vi "pwm_LED.vi"() -> ()   [LabVIEW 2011]
uses:
  <vilib>/LabVIEW Interface for Arduino/Type Defs/Pin Mode.ctl
  <vilib>/LabVIEW Interface for Arduino/LabVIEW Interface for Arduino.lvlib
panel:
  out "Waveform Chart":u8(graph)
  in  "stop":bool
  in  "PWM":u8(slide) scale=0.0..255.0
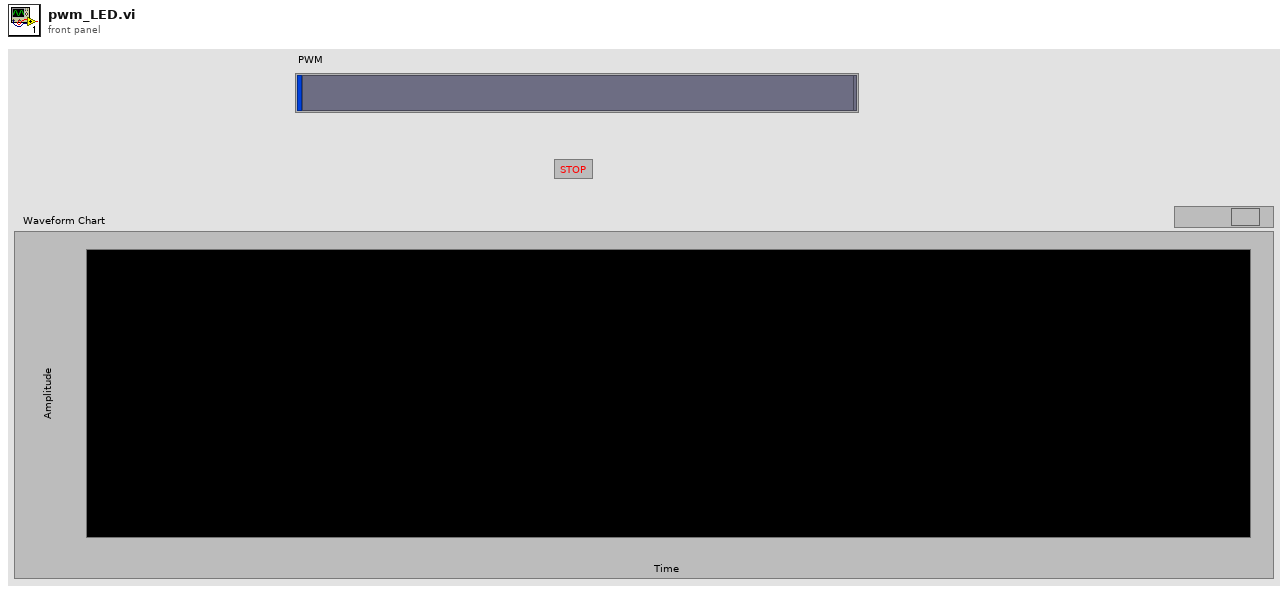
[diagram p1: front panel]
types:
  T1 = typedef "LabVIEW Interface for Arduino.lvlib/Arduino Resource.ctl" = cluster{"VISA resource":refnum<visa-resource-name>, "Board Type":T2, "Connection Type":enum8{"USB / Serial"}, "Bytes Per Packet (15)":u8}
  T2 = typedef "LabVIEW Interface for Arduino.lvlib/Board Type.ctl" = enum16{"Uno", "Dimuelanove w/Atmega 328", "Mega 2560"}
  T3 = typedef "LabVIEW Interface for Arduino.lvlib/Pin Mode.ctl" = enum8{"Input", "Output"}
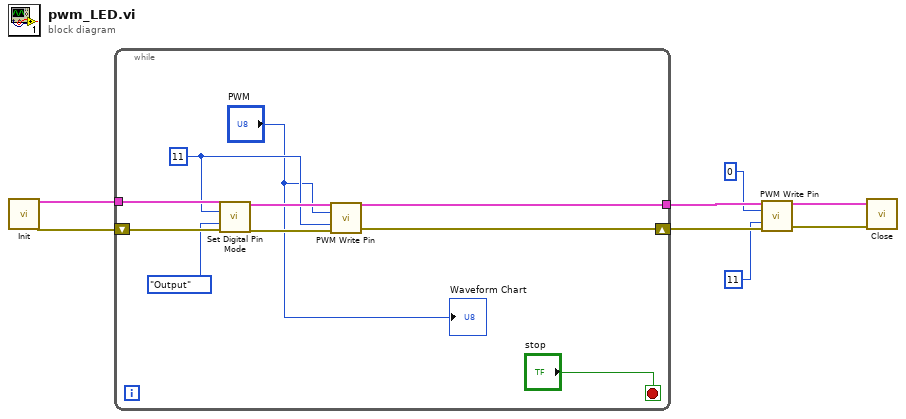
[diagram p0: block diagram]
diagram:
  n1 = call <vilib>:"Init.vi"() -> ("Arduino Resource"=w8:T1, "error out"=w3:errorcluster)  [unwired: 18 in]
  n2 = while {
    tunnel: w8 -> [w17]
    tunnel: [w15] -> w7
    shift-right: [w14] -> w4
    shift-left: w3 -> [w12]
    stop <- "stop" stop-if-true
    w10 = u8 11 ("Digital I/O Pin")
    n3 = call <vilib>:"Set Digital Pin Mode.vi"("Arduino Resource"=w17, "Digital I/O Pin"=w10, "Pin Mode (Input)"=Pin_Mode."Output", "error in"=w12) -> ("Arduino Resource"=w16:T1, "error out"=w13:errorcluster)  [unwired: 10 in]
    n4 = call <vilib>:"PWM Write Pin.vi"("Arduino Resource"=w16, "Duty Cycle (0 - 255)"="PWM", "PWM Pin (3)"=w10, "error in"=w13) -> ("Arduino Resource"=w15:T1, "error out"=w14:errorcluster)  [unwired: 10 in]
    "Waveform Chart" <- "PWM"
  }
  n5 = call <vilib>:"PWM Write Pin.vi"("Arduino Resource"=w7, "Duty Cycle (0 - 255)"=u8 0 ("PWM Pin (3)"), "PWM Pin (3)"=u8 11, "error in"=w4) -> ("Arduino Resource"=w6:T1, "error out"=w5:errorcluster)  [unwired: 10 in]
  n6 = call <vilib>:"Close.vi"("Arduino Resource"=w6, "error in"=w5) -> ()  [unwired: 13 in, 1 out]
